vi "main.vi"() -> ()   [LabVIEW 2018]
doc: "This example demonstrates the use of binary morphological reconstruction in the particle analysis. The example allows you to keep the particles completely inside the ROI, completely outside the ROI or on the ROI."
uses:
  <vilib>/vision/NI_Vision_Development_Module.lvlib
panel:
  out "标注后的图片路径":path
  out "标注图ROI2Mask":T1(plugin-control)
  out "反射图路径":path
  out "穿透图路径":path
  in  "Font, Size & Style":T2={"Desired Font (Application)"=enum."Application Font", "[User-specified Font]"={"Font Name"="", "Size"=12, "Strikeout?"=FALSE, "Italic?"=FALSE, "Underline?"=FALSE, "Outline?"=FALSE, "Shadow?"=FALSE, "Bold?"=FALSE, "Rotation Angle"=0.0}, "Horizontal Alignment"=0, "Vertical Alignment"=0} {"Horizontal Alignment" items=["Left", "Center", "Right"]; "Vertical Alignment" items=["Bottom", "Top", "Baseline"]}
  in  "Font, Size & Style 3":T2={"Desired Font (Application)"=enum."Application Font", "[User-specified Font]"={"Font Name"="", "Size"=12, "Strikeout?"=FALSE, "Italic?"=FALSE, "Underline?"=FALSE, "Outline?"=FALSE, "Shadow?"=FALSE, "Bold?"=FALSE, "Rotation Angle"=0.0}, "Horizontal Alignment"=0, "Vertical Alignment"=0} {"Vertical Alignment" items=["Bottom", "Top", "Baseline"]; "Horizontal Alignment" items=["Left", "Center", "Right"]; "[User-specified Font]"."Rotation Angle" format="%.2f"}
  out "总面积":i32
  out "ROI左上角坐标":cluster{i32, i32}
  out "透射图灰度表":u32[](graph)
  out "全图灰度级信息":T3 {"标准差" format="%.2f"; "均值" format="%.2f"; "相邻灰度级间隔" format="%.2f"; "起始灰度值" format="%.2f"; "最大值" format="%.2f"; "最小值" format="%.2f"}
  out "最大灰度值":sgl
  out "标注图":T1(plugin-control)
  out "写入数据库路径":path
  out "反射图灰度表":u32[](graph)
  out "反射图":T1(plugin-control)
  out "最大灰度值":sgl
  out "框数":dbl
  out "全图灰度级信息":T3 {"标准差" format="%.2f"; "均值" format="%.2f"; "相邻灰度级间隔" format="%.2f"; "起始灰度值" format="%.2f"; "最大值" format="%.2f"; "最小值" format="%.2f"}
  in  "评定报告生成":bool
  in  "部位":string
  in  "产品序号":string
  in  "测试人":string
  in  "预处理":bool
  in  "查看标注":bool
  in  "导入图像":bool
  in  "删除标注":bool
  in  "退出":bool
  in  "Font, Size & Style 2":T2={"Desired Font (Application)"=enum."Application Font", "[User-specified Font]"={"Font Name"="", "Size"=12, "Strikeout?"=FALSE, "Italic?"=FALSE, "Underline?"=FALSE, "Outline?"=FALSE, "Shadow?"=FALSE, "Bold?"=FALSE, "Rotation Angle"=0.0}, "Horizontal Alignment"=0, "Vertical Alignment"=0} {"Vertical Alignment" items=["Bottom", "Top", "Baseline"]; "Horizontal Alignment" items=["Left", "Center", "Right"]; "[User-specified Font]"."Rotation Angle" format="%.2f"}
  out "框组":T4(array[cluster])
  in  "Operation":enum16{"overlay rectangle"}(ring)
  # "穿透法图像"
  # "反射法图像"
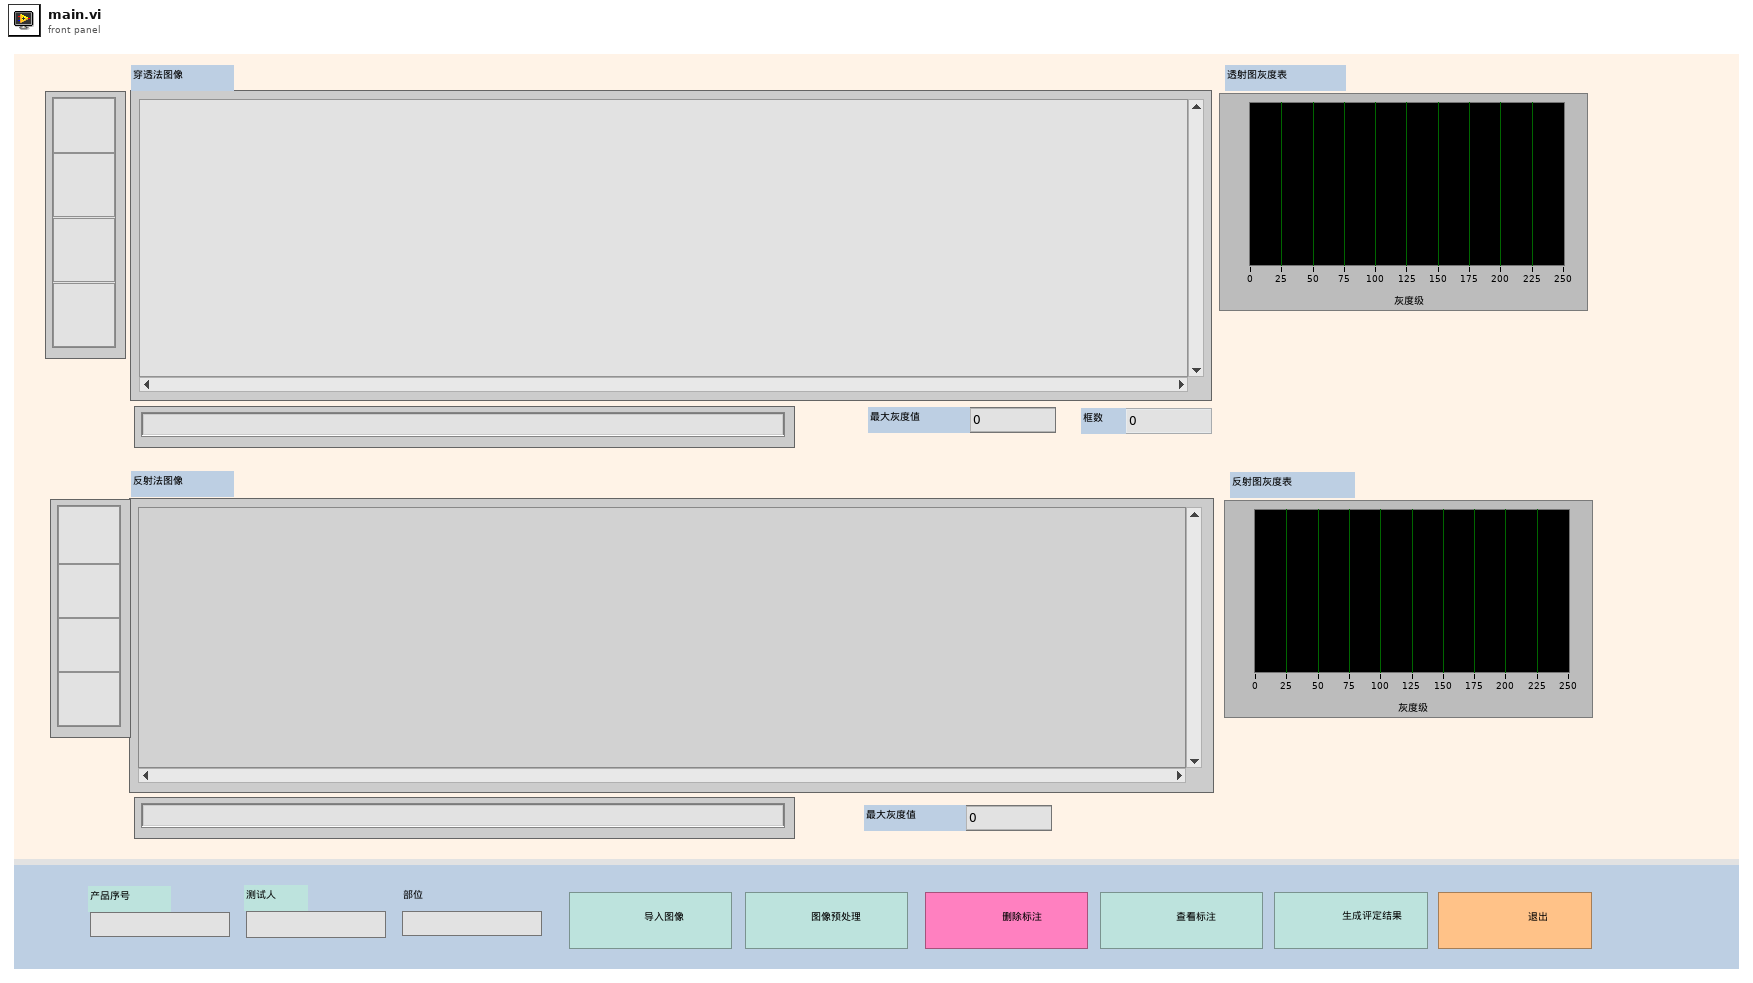
[diagram p1: front panel]
types:
  T1 = typedef "IMAQ Image.ctl" = refnum<image>
  T2 = cluster{"Desired Font (Application)":enum16{"User-specified Font", "Application Font", "System Font", "Dialog Font"}, "[User-specified Font]":cluster{"Font Name":string, "Size":i16, "Strikeout?":bool, "Italic?":bool, "Underline?":bool, "Outline?":bool, "Shadow?":bool, "Bold?":bool, "Rotation Angle":dbl}, "Horizontal Alignment":i16, "Vertical Alignment":i16}
  T3 = cluster{"histogram":u32[], "最小值":sgl, "最大值":sgl, "起始灰度值":sgl, "相邻灰度级间隔":sgl, "均值":sgl, "标准差":sgl, "像素面积":i32}
  T4 = cluster{"Global Rectangle":i32[], "Contours":cluster{"Contour Type":u32, "ROI Type":u32, "Points":i32[]}[]}[]
  T5 = typedef "Image Type" = u32
  T6 = cluster{"Global Rectangle":i32[], "Contours":cluster{"Contour Type":u32, "ROI Type":u32, "Points":i32[]}[]}
  T7 = cluster{"histogram":u32[], "Minimal Value":sgl, "Maximal Value":sgl, "Starting Value":sgl, "Interval Width":sgl, "Mean Value":sgl, "Standard  Variation":sgl, "Area (pixels)":i32}
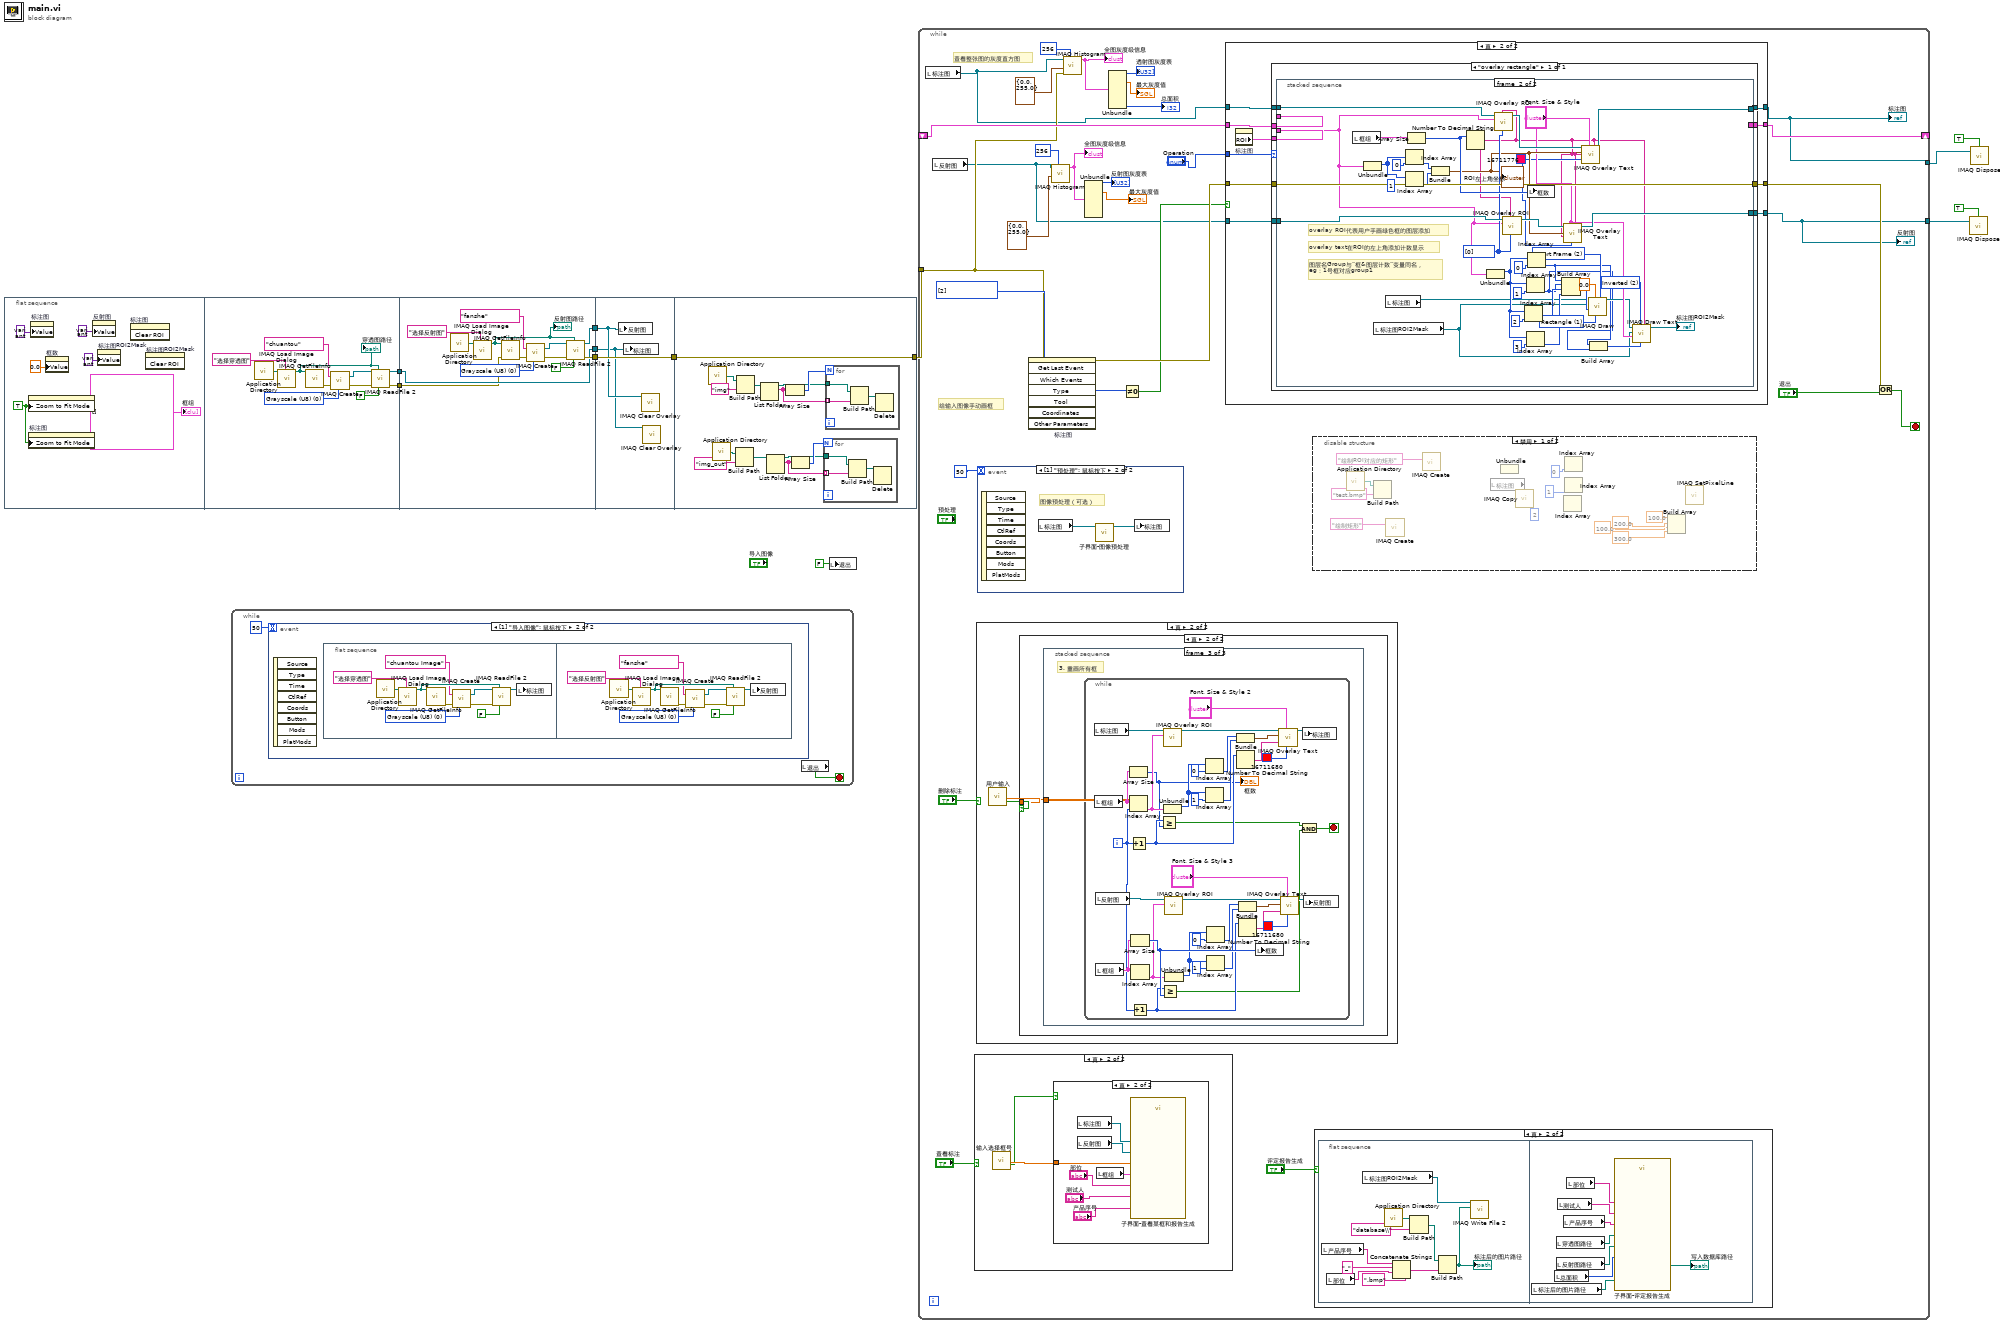
[diagram p0: block diagram]
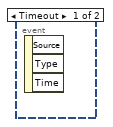
[diagram p2: hidden frame]
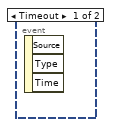
[diagram p5: hidden frame]
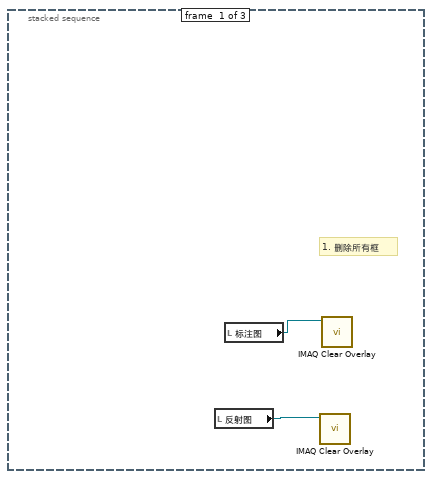
[diagram p10: hidden frame]
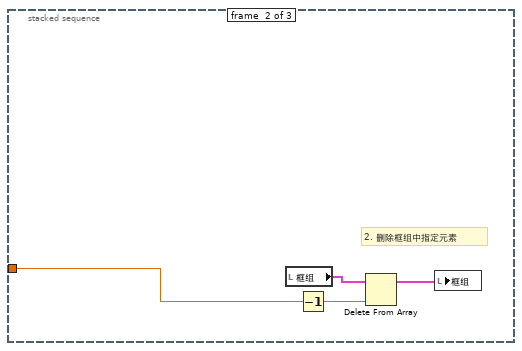
[diagram p11: hidden frame]
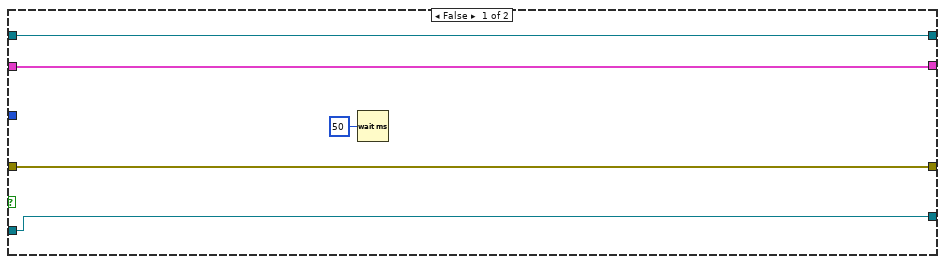
[diagram p12: hidden frame]
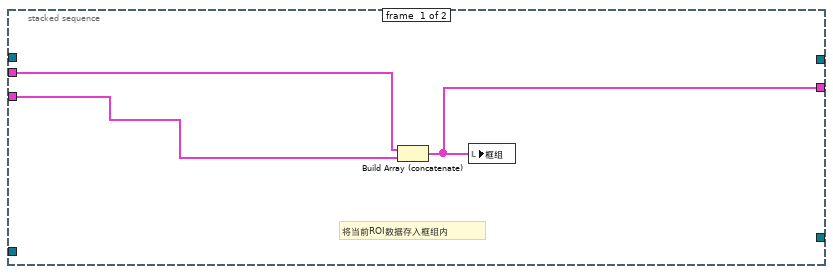
[diagram p13: hidden frame]
diagram:
  n1 = flat-sequence {
    tunnel: [w20] -> w9
    tunnel: [w19] -> w8
    tunnel: w9 -> [w32]
    tunnel: w8 -> [w33]
    tunnel: [w34] -> w7
    tunnel: [w33] -> w6
    tunnel: [w31] -> w5
    tunnel: w7 -> [w45]
    tunnel: w6 -> [w43]
    tunnel: w5 -> [w44]
    tunnel: [w45] -> w1
    tunnel: [w58] -> w12
    tunnel: w1 -> [w58]
    frame #0 {
      w17 = TRUE ("Zoom to Fit Mode")
      n2 = property on="反射图" class="ImageControl"("Zoom to Fit Mode"=w17) -> ()  [unwired: 2 in, 2 out]
      n3 = property on="标注图" class="ImageControl"("Zoom to Fit Mode"=w17) -> ()  [unwired: 2 in, 2 out]
      n4 = property on="标注图" class="ImageControl"("Value"=variant ("值")) -> ()  [unwired: 2 in, 2 out]
      n5 = property on="框数" class="DigNum (严格)"("Value"=0.0 ("标注框总数")) -> ()  [unwired: 2 in, 2 out]
      n6 = property on="反射图" class="ImageControl"("Value"=variant ("值")) -> ()  [unwired: 2 in, 2 out]
      n7 = property on="标注图ROI2Mask" class="ImageControl"("Value"=variant ("值")) -> ()  [unwired: 2 in, 2 out]
      n8 = invoke on="标注图" class="ImageControl" method="Clear ROI"() -> ()  [unwired: 3 in, 3 out]
      n9 = invoke on="标注图ROI2Mask" class="ImageControl" method="Clear ROI"() -> ()  [unwired: 3 in, 3 out]
      "框组" <- T4 [] ("框组")
    }
    frame #1 {
      w21 = T5 0 items=["Grayscale (U8)", "Grayscale (I16)", "Grayscale (SGL)", "Complex (CSG)", "RGB (U32)", "HSL (U32)", "RGB (U64)", "Grayscale (U16)"] ("Image Type")
      n10 = call <vilib>:"Application Directory.vi"() -> ("Application Directory"=w29:path)
      n11 = call "IMAQ Load Image Dialog"("Prompt"="选择穿透图" ("prompt"), "Start Path"=w29) -> ("Path"=w25:path)  [unwired: 7 in, 2 out]
      "穿透图路径" <- w25
      n12 = call "IMAQ GetFileInfo"("File Path"=w25) -> ("error out"=w26:errorcluster)  [unwired: 4 in, 6 out]
      n13 = call "IMAQ Create"("Image Name"="chuantou", "Image Type"=w21, "error in (no error)"=w26) -> ("New Image"=w27:T1, "error out"=w28:errorcluster)  [unwired: 2 in]
      n14 = call "IMAQ ReadFile 2"("Use File Path Image Type"=FALSE, "File Path"=w25, "error in (no error)"=w28, "Image"=w27) -> ("error out"=w20:errorcluster, "Image Out"=w19:T1)  [unwired: 3 in, 3 out]
    }
    frame #2 {
      w35 = T5 0 items=["Grayscale (U8)", "Grayscale (I16)", "Grayscale (SGL)", "Complex (CSG)", "RGB (U32)", "HSL (U32)", "RGB (U64)", "Grayscale (U16)"] ("Image Type")
      n15 = call <vilib>:"Application Directory.vi"() -> ("Application Directory"=w42:path)
      n16 = call "IMAQ Load Image Dialog"("Prompt"="选择反射图" ("prompt"), "Start Path"=w42) -> ("Path"=w30:path)  [unwired: 7 in, 2 out]
      "反射图路径" <- w30
      n17 = call "IMAQ GetFileInfo"("error in (no error)"=w32, "File Path"=w30) -> ("error out"=w39:errorcluster)  [unwired: 3 in, 6 out]
      n18 = call "IMAQ Create"("Image Name"="fanshe", "Image Type"=w35, "error in (no error)"=w39) -> ("New Image"=w40:T1, "error out"=w41:errorcluster)  [unwired: 2 in]
      n19 = call "IMAQ ReadFile 2"("Use File Path Image Type"=FALSE, "File Path"=w30, "error in (no error)"=w41, "Image"=w40) -> ("error out"=w34:errorcluster, "Image Out"=w31:T1)  [unwired: 3 in, 3 out]
    }
    frame #3 {
      n20 = local write "反射图"(w44) -> ()
      n21 = local write "标注图"(w43) -> ()
      n22 = call "IMAQ Clear Overlay"("Image"=w44) -> ()  [unwired: 9 in, 2 out]
      n23 = call "IMAQ Clear Overlay"("Image"=w43) -> ()  [unwired: 9 in, 2 out]
    }
    frame #4 {
      n24 = call <vilib>:"Application Directory.vi"() -> ("Application Directory"=w54:path)
      n25 = call <vilib>:"Application Directory.vi"() -> ("Application Directory"=w48:path)
      n26 = Build Path(base path=w48, name or relative path="img_out" ("名称或相对路径")) -> (appended path=w49:path)
      n27 = Build Path(base path=w54, name or relative path="img" ("名称或相对路径")) -> (appended path=w55:path)
      n28 = List Folder(path=w55) -> (path out=w53:path, filenames=w57:string[])  [unwired: 3 in, 2 out]
      n29 = List Folder(path=w49) -> (path out=w47:path, filenames=w51:string[])  [unwired: 3 in, 2 out]
      n30 = Array Size(array=w57) -> (size(s)=w56:i32)
      n31 = Array Size(array=w51) -> (size(s)=w50:i32)
      n32 = for {
        N: w50 -> [_]
        tunnel: w47 -> [w60]
        tunnel: w51 -> [w59] mode=indexing
        n33 = Build Path(base path=w60, name or relative path=w59) -> (appended path=w61:path)
        n34 = Delete(path (use dialog)=w61) -> ()  [unwired: 4 in, 3 out]
      }
      n35 = for {
        N: w56 -> [_]
        tunnel: w53 -> [w63]
        tunnel: w57 -> [w62] mode=indexing
        n36 = Build Path(base path=w63, name or relative path=w62) -> (appended path=w64:path)
        n37 = Delete(path (use dialog)=w64) -> ()  [unwired: 4 in, 3 out]
      }
    }
  }
  n38 = while {
    stop <- w65 stop-if-true
    n39 = event shown="[1] \"导入图像\": 鼠标按下" {
      selector: _ -> [_ _]
      dyn-events: _ -> [_ _]
      timeout: 50 -> [_ _]
      event Timeout {
        n40 = event-data() -> ()  [unwired: 1 in, 3 out]
      }
      event "导入图像": Mouse Down {
        n41 = event-data() -> ()  [unwired: 1 in, 8 out]
        n42 = flat-sequence {
          frame #0 {
            w68 = T5 0 items=["Grayscale (U8)", "Grayscale (I16)", "Grayscale (SGL)", "Complex (CSG)", "RGB (U32)", "HSL (U32)", "RGB (U64)", "Grayscale (U16)"] ("Image Type")
            n43 = call <vilib>:"Application Directory.vi"() -> ("Application Directory"=w76:path)
            n44 = call "IMAQ Load Image Dialog"("Prompt"="选择穿透图" ("prompt"), "Start Path"=w76) -> ("Path"=w72:path)  [unwired: 7 in, 2 out]
            n45 = call "IMAQ GetFileInfo"("File Path"=w72) -> ("error out"=w73:errorcluster)  [unwired: 4 in, 6 out]
            n46 = call "IMAQ Create"("Image Name"="chuantou Image", "Image Type"=w68, "error in (no error)"=w73) -> ("New Image"=w74:T1, "error out"=w75:errorcluster)  [unwired: 2 in]
            n47 = call "IMAQ ReadFile 2"("Use File Path Image Type"=FALSE, "File Path"=w72, "error in (no error)"=w75, "Image"=w74) -> ("Image Out"=w67:T1)  [unwired: 3 in, 4 out]
            n48 = local write "标注图"(w67) -> ()
          }
          frame #1 {
            w80 = T5 0 items=["Grayscale (U8)", "Grayscale (I16)", "Grayscale (SGL)", "Complex (CSG)", "RGB (U32)", "HSL (U32)", "RGB (U64)", "Grayscale (U16)"] ("Image Type")
            n49 = call <vilib>:"Application Directory.vi"() -> ("Application Directory"=w82:path)
            n50 = call "IMAQ Load Image Dialog"("Prompt"="选择反射图" ("prompt"), "Start Path"=w82) -> ("Path"=w86:path)  [unwired: 7 in, 2 out]
            n51 = call "IMAQ GetFileInfo"("File Path"=w86) -> ("error out"=w85:errorcluster)  [unwired: 4 in, 6 out]
            n52 = call "IMAQ Create"("Image Name"="fanshe", "Image Type"=w80, "error in (no error)"=w85) -> ("New Image"=w84:T1, "error out"=w83:errorcluster)  [unwired: 2 in]
            n53 = call "IMAQ ReadFile 2"("Use File Path Image Type"=FALSE, "File Path"=w86, "error in (no error)"=w83, "Image"=w84) -> ("Image Out"=w77:T1)  [unwired: 3 in, 4 out]
            n54 = local write "反射图"(w77) -> ()
          }
        }
      }
    }
    n55 = local read "退出"() -> (w65:bool)
  }
  n56 = local write "退出"(FALSE ("退出")) -> ()
  n57 = while {
    shift-right: [w109] -> _
    shift-left: _ -> [w108]
    tunnel: w12 -> [w107]
    tunnel: [w91] -> w10
    tunnel: [w92] -> w3
    stop <- w111 stop-if-true
    (unwired) "_" ("名称或相对路径")
    (unwired) ".docx" ("名称或相对路径")
    w114 = i32[] [2] items=["No Event"=0, "Click Event"=1, "Draw Event"=2, "Size Event"=4, "Scroll Event"=5, "Double Click Event"=8] ("Which Events")
    # "给输入图像手动画框"
    # "查看整张图的灰度直方图"
    n58 = local read "标注图"() -> (w93:T1)
    n59 = local read "反射图"() -> (w94:T1)
    n60 = case shown="真" "查看标注" {
      frame False {
      }
      frame True {
        n61 = call "输入选择框号"() -> ("框号"=w148:dbl, "确定"=w147:bool)  [unwired: 17 in, 1 out]
        n62 = case shown="真" w147 {
          tunnel: w148 -> [_ w155]
          frame False {
            # "用户取消操作"
          }
          frame True {
            n63 = local read "标注图"() -> (w152:T1)
            n64 = local read "反射图"() -> (w153:T1)
            n65 = local read "框组"() -> (w154:T4)
            n66 = call "子界面-查看某框和报告生成.vi"("测试人"="测试人", "标注图"=w152, "部位"="部位", "产品序号"="产品序号", "反射图"=w153, "框组"=w154, "框号"=w155) -> ()  [unwired: 3 in]
          }
        }
      }
    }
    n67 = case shown="真" "删除标注" {
      frame False {
      }
      frame True {
        n68 = call "用户输入"() -> ("框号"=w156:dbl, "确定"=w157:bool)  [unwired: 17 in, 1 out]
        n69 = case shown="真" w157 {
          tunnel: w156 -> [_ w158]
          frame False {
            # "用户取消操作"
          }
          frame True {
            n70 = stacked-sequence {
              tunnel: w158 -> [_ w163 _]
              frame #0 {
                # "1. 删除所有框"
                n71 = local read "反射图"() -> (w159:T1)
                n72 = local read "标注图"() -> (w160:T1)
                n73 = call "IMAQ Clear Overlay"("Image"=w159) -> ()  [unwired: 9 in, 2 out]
                n74 = call "IMAQ Clear Overlay"("Image"=w160) -> ()  [unwired: 9 in, 2 out]
              }
              frame #1 {
                # "2. 删除框组中指定元素"
                n75 = local read "框组"() -> (w164:T4)
                n76 = Decrement(x=w163) -> (x-1=w162:dbl)
                n77 = Delete From Array(array=w164, index=w162) -> (array with subset deleted=w161:T4)  [unwired: 1 in, 1 out]
                n78 = local write "框组"(w161) -> ()
              }
              frame #2 {
                # "3. 重画所有框"
                n79 = while {
                  i -> [w169]
                  stop <- w166 stop-if-true
                  n80 = local read "标注图"() -> (w200:T1)
                  n81 = local read "框组"() -> (w194:T4)
                  n82 = local read "反射图"() -> (w170:T1)
                  n83 = local read "框组"() -> (w176:T4)
                  n84 = Array Size(array=w194) -> (size(s)=w185:i32)
                  "框数" <- w185
                  n85 = Index Array(array=w194, index=w169) -> (element=w187:T6)
                  n86 = Increment(x=w169) -> (x+1=w199:i32)
                  n87 = Array Size(array=w176) -> (size(s)=w184:i32)
                  n88 = Index Array(array=w176) -> (element=w183:T6)  [unwired: 1 in]
                  n89 = Increment(x=w169) -> (x+1=w171:i32)
                  n90 = Greater Or Equal?(x=w199, y=w185) -> (x >= y?=w168:bool)
                  n91 = Greater Or Equal?(x=w171, y=w184) -> (x >= y?=w167:bool)
                  n92 = call "IMAQ Overlay ROI"("ROI Descriptor"=w187, "Image"=w200) -> ("Image Out"=w196:T1)  [unwired: 8 in, 1 out]
                  n93 = Unbundle(w187) -> ("Global Rectangle"=w190:i32[])  [unwired: 1 out]
                  n94 = call "IMAQ Overlay ROI"("ROI Descriptor"=w183, "Image"=w170) -> ("Image Out"=w174:T1)  [unwired: 8 in, 1 out]
                  n95 = Unbundle(w183) -> ("Global Rectangle"=w180:i32[])  [unwired: 1 out]
                  n96 = Index Array(array=w190, index=0 ("索引")) -> (element=w191:i32)
                  n97 = Index Array(array=w190, index=1 ("索引")) -> (element=w192:i32)
                  n98 = Index Array(array=w180, index=0 ("索引")) -> (element=w179:i32)
                  n99 = Index Array(array=w180, index=1 ("索引")) -> (element=w178:i32)
                  n100 = Bundle(w191, w192) -> (w189:cluster{i32, i32})  [unwired: 1 in]
                  n101 = Number To Decimal String(number=w199) -> (decimal integer string=w197:string)  [unwired: 1 in]
                  n102 = Bundle(w179, w178) -> (w181:cluster{i32, i32})  [unwired: 1 in]
                  n103 = Number To Decimal String(number=w171) -> (decimal integer string=w173:string)  [unwired: 1 in]
                  n104 = local write "框数"(w184) -> ()
                  n105 = call "IMAQ Overlay Text"("Text Color (black)"=u32 16711680, "Font, Size & Style"="Font, Size & Style 2", "String"=w197, "Origin"=w189, "Image"=w196) -> ("Image Out"=w195:T1)  [unwired: 5 in, 1 out]
                  n106 = call "IMAQ Overlay Text"("Text Color (black)"=u32 16711680, "Font, Size & Style"="Font, Size & Style 3", "String"=w173, "Origin"=w181, "Image"=w174) -> ("Image Out"=w175:T1)  [unwired: 5 in, 1 out]
                  n107 = And(x=w168, y=w167) -> (x .and. y?=w166:bool)
                  n108 = local write "标注图"(w195) -> ()
                  n109 = local write "反射图"(w175) -> ()
                }
              }
            }
          }
        }
      }
    }
    n110 = event shown="[1] \"预处理\": 鼠标按下" {
      selector: _ -> [_ _]
      dyn-events: _ -> [_ _]
      timeout: 50 -> [_ _]
      event Timeout {
        n111 = event-data() -> ()  [unwired: 1 in, 3 out]
      }
      event "预处理": Mouse Down {
        # "图像预处理（可选）"
        n112 = event-data() -> ()  [unwired: 1 in, 8 out]
        n113 = local read "标注图"() -> (w146:T1)
        n114 = call "子界面-图像预处理.vi"("原图"=w146) -> ("处理后"=w145:T1)  [unwired: 10 in]
        n115 = local write "标注图"(w145) -> ()
      }
    }
    n116 = invoke on="标注图" class="ImageControl" method="Get Last Event"(error in=w107, "Which Events"=w114) -> (error out=w113:errorcluster, "Type"=w115:i32)  [unwired: 6 in, 6 out]
    n117 = call "IMAQ Histogram"("Number of Classes"=256, "Interval Range"=cluster{"Minimum":sgl, "Maximum":sgl} {"Minimum"=0.0, "Maximum"=255.0}, "Image"=w94) -> ("Histogram Report"=w96:T7)  [unwired: 7 in, 1 out]
    "全图灰度级信息" <- w96
    n118 = call "IMAQ Histogram"("Number of Classes"=256, "error in (no error)"=w107, "Interval Range"=cluster{"Minimum":sgl, "Maximum":sgl} {"Minimum"=0.0, "Maximum"=255.0}, "Image"=w93) -> ("Histogram Report"=w98:T7)  [unwired: 6 in, 1 out]
    "全图灰度级信息" <- w98
    n119 = Unbundle(w96) -> ("histogram"=→"反射图灰度表":u32[], "Maximal Value"=→"最大灰度值":sgl)  [unwired: 6 out]
    n120 = Unbundle(w98) -> ("histogram"=→"透射图灰度表":u32[], "Maximal Value"=→"最大灰度值":sgl, "Area (pixels)"=→"总面积":i32)  [unwired: 5 out]
    n121 = Not Equal To 0?(x=w115) -> (x != 0?=w110:bool)
    n122 = case shown="真" w110 {
      tunnel: w93 -> [w205 w215]
      tunnel: [w205 w214] -> w91
      tunnel: "Operation" -> [_ w212]
      tunnel: w113 -> [w204 w211]
      tunnel: [w204 w210] -> w112
      tunnel: [w202 w209] -> w109
      tunnel: w108 -> [w202 w208]
      tunnel: w94 -> [w201 w207]
      tunnel: [w201 w206] -> w92
      frame False {
        n123 = Wait (ms)(milliseconds to wait=u32 50) -> ()  [unwired: 1 out]
      }
      frame True {
        n124 = property on="标注图" class="ImageControl"() -> ("ROI"=w213:T6)  [unwired: 2 in, 2 out]
        n125 = case shown="\"overlay rectangle\"" w212 {
          tunnel: w215 -> [w222]
          tunnel: w213 -> [w220]
          tunnel: [w221] -> w214
          tunnel: w211 -> [w223]
          tunnel: [w223] -> w210
          tunnel: [w219] -> w209
          tunnel: w208 -> [w218]
          tunnel: w207 -> [w217]
          tunnel: [w216] -> w206
          frame "overlay rectangle" {
            n126 = stacked-sequence {
              tunnel: w222 -> [_ w250]
              tunnel: [_ w257] -> w221
              tunnel: w220 -> [w226 w249]
              tunnel: [w224 _] -> w219
              tunnel: w218 -> [w225 _]
              tunnel: w217 -> [_ w255]
              tunnel: [_ w254] -> w216
              frame #0 {
                # "将当前ROI数据存入框组内"
                n127 = Build Array (concatenate)(w225, w226) -> (w224:T4)
                n128 = local write "框组"(w224) -> ()
              }
              frame #1 {
                w228 = 2 items=["White", "Black", "Inverted", "Black on White", "White on Black"] ("Color")
                w237 = u16 2 items=["Frame", "Paint", "Invert Frame", "Invert Paint"] ("Draw Mode")
                w240 = u16 1 items=["Line", "Rectangle", "Oval"] ("Shape to draw")
                w252 = u32[] [0] ("Colors (Green)")
                w235 = u32 16711776 ("Text Color (black)")
                # "图层名Group与“框&图层计数”变量同名，\neg：1号框对应group1"
                # "overlay text在ROI的左上角添加计数显示"
                # "overlay ROI代表用户手画绿色框的图层添加"
                n129 = local read "框组"() -> (w260:T4)
                n130 = Unbundle(w249) -> ("Global Rectangle"=w263:i32[])  [unwired: 1 out]
                n131 = local read "标注图ROI2Mask"() -> (w227:T1)
                n132 = local read "标注图"() -> (w239:T1)
                n133 = Index Array(array=w263, index=0 ("索引")) -> (element=w262:i32)
                n134 = Index Array(array=w263, index=1 ("索引")) -> (element=w261:i32)
                n135 = Array Size(array=w260) -> (size(s)=w256:i32)
                n136 = Bundle(w262, w261) -> (w251:cluster{i32, i32})  [unwired: 1 in]
                "ROI左上角坐标" <- w251
                n137 = Number To Decimal String(number=w256) -> (decimal integer string=w234:string)  [unwired: 1 in]
                n138 = Unbundle(w249) -> ("Global Rectangle"=w244:i32[])  [unwired: 1 out]
                n139 = call "IMAQ Overlay ROI"("Colors (Green)"=w252, "Group"=w234, "ROI Descriptor"=w249, "Image"=w250) -> ("Image Out"=w264:T1)  [unwired: 6 in, 1 out]
                n140 = call "IMAQ Overlay ROI"("Colors (Green)"=w252, "Group"=w234, "ROI Descriptor"=w249, "Image"=w255) -> ("Image Out"=w253:T1)  [unwired: 6 in, 1 out]
                n141 = Index Array(array=w244, index=2 ("索引")) -> (element=w243:i32)
                n142 = Index Array(array=w244, index=1 ("索引")) -> (element=w230:i32)
                n143 = Index Array(array=w244, index=3 ("索引")) -> (element=w242:i32)
                n144 = local write "框数"(w256) -> ()
                n145 = Index Array(array=w244, index=0 ("索引")) -> (element=w231:i32)
                n146 = Build Array(w231, w230, w243, w242) -> (w241:i32[])
                n147 = call "IMAQ Overlay Text"("Group"=w234, "Text Color (black)"=w235, "Font, Size & Style"="Font, Size & Style", "String"=w234, "Origin"=w251, "Image"=w253) -> ("Image Out"=w254:T1)  [unwired: 4 in, 1 out]
                n148 = call "IMAQ Overlay Text"("Group"=w234, "Text Color (black)"=w235, "Font, Size & Style"="Font, Size & Style", "String"=w234, "Origin"=w251, "Image"=w264) -> ("Image Out"=w257:T1)  [unwired: 4 in, 1 out]
                n149 = call "IMAQ Draw"("Draw Mode"=w237, "Shape to draw"=w240, "Pixel Color"=sgl 0.0, "Coordinates"=w241, "Image Dst"=w227, "Image Src"=w239) -> ("Image Dst Out"=w233:T1)  [unwired: 4 in, 1 out]
                n150 = Build Array(w231, w230) -> (w229:i32[])
                n151 = call "IMAQ Draw Text"("String"=w234, "Insertion Point"=w229, "Color"=w228, "Font, Size & Style"="Font, Size & Style", "Image Dst"=w227, "Image Src"=w233) -> ("Image Dst Out"=→"标注图ROI2Mask":T1)  [unwired: 2 in, 3 out]
              }
            }
          }
        }
      }
    }
    "标注图" <- w91
    "反射图" <- w92
    n152 = disable-structure shown="禁用" {
      frame Disabled {
        (unwired) 2 ("索引")
        n153 = call <vilib>:"Application Directory.vi"() -> ("Application Directory"=w120:path)
        n154 = Build Path(base path=w120, name or relative path="test.bmp" ("名称或相对路径")) -> ()  [unwired: 1 out]
        n155 = call "IMAQ Create"("Image Name"="绘制矩形") -> ()  [unwired: 4 in, 2 out]
        n156 = call "IMAQ Create"("Image Name"="绘制ROI对应的矩形") -> ()  [unwired: 4 in, 2 out]
        n157 = local read "标注图"() -> ()  [unwired: 1 out]
        n158 = Unbundle() -> ()  [unwired: 1 in, 2 out]
        n159 = call "IMAQ Copy"() -> ()  [unwired: 6 in, 2 out]
        n160 = Index Array() -> ()  [unwired: 2 in, 1 out]
        n161 = Index Array(index=0 ("索引")) -> ()  [unwired: 1 in, 1 out]
        n162 = Index Array(index=1 ("索引")) -> ()  [unwired: 1 in, 1 out]
        n163 = Build Array(100.0 ("元素"), 200.0 ("元素"), 100.0 ("元素"), 300.0 ("元素")) -> ()  [unwired: 1 out]
        n164 = call "IMAQ SetPixelLine"() -> ()  [unwired: 10 in, 2 out]
      }
      frame Enabled {
      }
    }
    n165 = case shown="真" "评定报告生成" {
      frame False {
      }
      frame True {
        n166 = flat-sequence {
          frame #0 {
            n167 = local read "产品序号"() -> (w130:string)
            n168 = local read "部位"() -> (w128:string)
            n169 = local read "标注图ROI2Mask"() -> (w136:T1)
            n170 = call <vilib>:"Application Directory.vi"() -> ("Application Directory"=w134:path)
            n171 = Concatenate Strings(w130, "_" ("名称或相对路径"), w128, ".bmp" ("名称或相对路径")) -> (w133:string)
            n172 = Build Path(base path=w134, name or relative path="database\\" ("名称或相对路径")) -> (appended path=w135:path)
            n173 = Build Path(base path=w135, name or relative path=w133) -> (appended path=w127:path)
            "标注后的图片路径" <- w127
            n174 = call-poly "IMAQ Write File 2"("File Path"=w127, "Image"=w136) -> ()  [unwired: 8 in, 2 out]
          }
          frame #1 {
            n175 = local read "标注后的图片路径"() -> (w137:path)
            n176 = local read "总面积"() -> (w143:i32)
            n177 = local read "穿透图路径"() -> (w139:path)
            n178 = local read "反射图路径"() -> (w138:path)
            n179 = local read "测试人"() -> (w141:string)
            n180 = local read "产品序号"() -> (w140:string)
            n181 = local read "部位"() -> (w142:string)
            n182 = call "子界面-评定报告生成.vi"("反射图路径"=w138, "标注后的图片路径"=w137, "总面积"=w143, "部位"=w142, "穿透图路径"=w139, "测试人"=w141, "产品序号"=w140) -> ("写入数据库路径"=→"写入数据库路径":path)  [unwired: 3 in]
          }
        }
      }
    }
    n183 = Or(x=w112, y="退出") -> (x .or. y?=w111:bool)
    n184 = call <vilib>:"Application Directory.vi"() -> ()  [unwired: 1 out]
  }
  n185 = call "IMAQ Dispose"("All Images? (No)"=TRUE, "Image"=w3) -> ()  [unwired: 1 in, 4 out]
  n186 = call "IMAQ Dispose"("All Images? (No)"=TRUE, "Image"=w10) -> ()  [unwired: 1 in, 4 out]
